vi "M2p_AD+DA_Std_Sync.vi"() -> ()   [LabVIEW 2015]
uses:
  spcm_library/spcm_gui_m2p.llb/element_m2p_ad_std.ctl
  spcm_library/spcm_gui_m2p.llb/element_m2p_ai_channel.ctl
  spcm_library/spcm_gui_common.llb/element_mode.ctl
  spcm_library/spcm_gui_m2p.llb/element_m2p_clock.ctl
  spcm_library/spcm_gui_m2p.llb/element_m2p_ai_trigger.ctl
  spcm_library/spcm_gui_m2p.llb/element_m2p_ai_multi_purpose_io.ctl
  spcm_library/spcm_gui_m2p.llb/element_m2p_da_std.ctl
  spcm_library/spcm_gui_m2p.llb/element_m2p_ao_channel.ctl
  spcm_library/spcm_gui_common.llb/element_mode_out.ctl
  spcm_library/spcm_gui_m2p.llb/element_m2p_ao_trigger.ctl
  spcm_library/spcm_gui_m2p.llb/element_m2p_ao_multi_purpose_io.ctl
  spcm_library/spcm_gui_common.llb/element_devices.ctl
  spcm_library/spcm_gui_common.llb/element_states_io_sync.ctl
panel:
  in  "Waveform":cluster{"Waveform":u16, "Ampl / %":dbl}={"Waveform"=0, "Ampl / %"=100.0} {"Waveform" items=["Sine", "Square", "Ramp"]}
  out "Display Data":sgl[][](graph)
  in  "Devices":T1 {"Device" items=["Card", "digitizerNETBOX"]}
  in  "Tab Control":enum32{"AD Settings", "DA Settings"}(tab)
  in  "Array AD Settings":T2[](array[typedef])=[{"AI Channel 0"={"Enable"=TRUE, "Input Range "=2, "Termination"=0, "Input Type"=0, "Offset"=0}, "AI Channel 1"={"Enable"=TRUE, "Input Range "=2, "Termination"=0, "Input Type"=0, "Offset"=0}, "AI Channel 2"={"Enable"=TRUE, "Input Range "=2, "Termination"=0, "Input Type"=0, "Offset"=0}, "AI Channel 3"={"Enable"=TRUE, "Input Range "=2, "Termination"=0, "Input Type"=0, "Offset"=0}, "AI Channel 4"={"Enable"=TRUE, "Input Range "=2, "Termination"=0, "Input Type"=0, "Offset"=0}, "AI Channel 5"={"Enable"=TRUE, "Input Range "=2, "Termination"=0, "Input Type"=0, "Offset"=0}, "AI Channel 6"={"Enable"=TRUE, "Input Range "=2, "Termination"=0, "Input Type"=0, "Offset"=0}, "AI Channel 7"={"Enable"=TRUE, "Input Range "=2, "Termination"=0, "Input Type"=0, "Offset"=0}, "Mode Setup"={"Mode"=0, "Mem"=16384, "Seg"=1024, "Post"=8192, "Pre"=32, "ABA"=16}, "Clock Settings"={"Clock Mode"=0, "Sampling Rate (kHz)"=10000.0, "Clock Output"=FALSE, "Termination"=FALSE, "Ref. Clock (MHz)"=10.0, "Threshold (mV)"=1500}, "Trigger Settings"={"Trigger Source"=0, "External Trigger"=0, "Level 0 Ext"=1500, "Ext Trig Term"=FALSE, "Channel Trigger"=1, "Level 0 Ch"=0, "Level 1 Ch"=0, "Trigger Delay (Samples)"=0}, "Multi Purpose IO Lines"={"X0 Mode"=0, "X1 Mode"=0, "X2 Mode"=0, "X3 Mode"=0, "X0 ASync Send Pulse"=FALSE, "X1 ASync Send Pulse"=FALSE, "X2 ASync Send Pulse"=FALSE, "X3 ASync Send Pulse"=FALSE, "X1 Trigger Mode"=0, "X2 Trigger Mode"=0, "X3 Trigger Mode"=0, "X1 Pulsewidth"=0, "X2 Pulsewidth"=0, "X3 Pulsewidth"=0, "ASync Read Button"=FALSE, "ASync Read"=0, "AI"=FALSE}}] {"Multi Purpose IO Lines"."X3 Mode" items=["Disable", "Asynchronous Out", "Asynchronous In", "Trigger Out", "Trigger In", "Clock Out", "Digital In", "Show Run State", "Show Arm State", "Show Sync Arm State"]; "Multi Purpose IO Lines"."X2 Mode" items=["Disable", "Asynchronous Out", "Asynchronous In", "Trigger Out", "Trigger In", "Clock Out", "Digital In", "Show Run State", "Show Arm State", "Show Sync Arm State"]; "Multi Purpose IO Lines"."X3 Trigger Mode" items=["Pos. Edge", "Neg. Edge", "Any Edge", "High Level", "Low Level", "PW Long Pos.", "PW Long Neg.", "PW Short Pos.", "PW Short Neg."]; "Multi Purpose IO Lines"."X2 Trigger Mode" items=["Pos. Edge", "Neg. Edge", "Any Edge", "High Level", "Low Level", "PW Long Pos.", "PW Long Neg.", "PW Short Pos.", "PW Short Neg."]; "Multi Purpose IO Lines"."X1 Trigger Mode" items=["Pos. Edge", "Neg. Edge", "Any Edge", "High Level", "Low Level", "PW Long Pos.", "PW Long Neg.", "PW Short Pos.", "PW Short Neg."]; "Multi Purpose IO Lines"."X1 Mode" items=["Disable", "Asynchronous Out", "Asynchronous In", "Trigger Out", "Trigger In", "Clock Out", "Digital In", "Show Run State", "Show Arm State", "Show Sync Arm State"]; "Multi Purpose IO Lines"."X0 Mode" items=["Disable", "Asynchronous Out", "Trigger Out", "Clock Out", "Show Run State", "Show Arm State", "Show Sync Arm State"]; "Trigger Settings"."Channel Trigger" items=["None", "Pos. Edge", "Neg. Edge", "Any Edge", "Pos. Rearm", "Neg. Rearm", "Enter Window", "Leave Window", "In Win", "Out Win"]; "Trigger Settings"."External Trigger" items=["None", "Pos. Edge", "Neg. Edge", "Any Edge", "High Level", "Low Level"]; "Trigger Settings"."Trigger Source" items=["Software Trigger", "External Trigger", "Channel 0 Trigger", "Channel 1 Trigger", "Channel 2 Trigger", "Channel 3 Trigger", "Channel 4 Trigger", "Channel 5 Trigger", "Channel 6 Trigger", "Channel 7 Trigger"]; "Trigger Settings"."Trigger Delay (Samples)" max=65535 step=1; "Clock Settings"."Threshold (mV)" min=-5000 max=5000; "Clock Settings"."Clock Mode" items=["Internal Clock Quartz", "External Clock", "External Reference Clock"]; "Clock Settings"."Ref. Clock (MHz)" min=0.0 max=125000.0; "Clock Settings"."Sampling Rate (kHz)" min=1.0 max=5000000.0; "Mode Setup"."Mode" items=["Singleshot", "Multiple Recording", "Gated Sampling", "ABA Mode"]; "Mode Setup"."ABA" min=2 max=65535 step=1; "Mode Setup"."Post" min=4 step=4; "Mode Setup"."Mem" min=8 step=4; "Mode Setup"."Pre" min=4 max=8176 step=4; "Mode Setup"."Seg" min=8 step=4; "AI Channel 7"."Input Type" items=["Single-ended", "Differential"]; "AI Channel 7"."Termination" items=["1 MOhm", "50 Ohm"]; "AI Channel 7"."Input Range" items=["±200 mV", "±500 mV", "±1000 mV", "±2000 mV", "±5000 mV", "±10000 mV"]; "AI Channel 6"."Input Type" items=["Single-ended", "Differential"]; "AI Channel 6"."Termination" items=["1 MOhm", "50 Ohm"]; "AI Channel 6"."Input Range" items=["±200 mV", "±500 mV", "±1000 mV", "±2000 mV", "±5000 mV", "±10000 mV"]; "AI Channel 5"."Input Type" items=["Single-ended", "Differential"]; "AI Channel 5"."Termination" items=["1 MOhm", "50 Ohm"]; "AI Channel 5"."Input Range" items=["±200 mV", "±500 mV", "±1000 mV", "±2000 mV", "±5000 mV", "±10000 mV"]; "AI Channel 4"."Input Type" items=["Single-ended", "Differential"]; "AI Channel 4"."Termination" items=["1 MOhm", "50 Ohm"]; "AI Channel 4"."Input Range" items=["±200 mV", "±500 mV", "±1000 mV", "±2000 mV", "±5000 mV", "±10000 mV"]; "AI Channel 3"."Input Type" items=["Single-ended", "Differential"]; "AI Channel 3"."Termination" items=["1 MOhm", "50 Ohm"]; "AI Channel 3"."Input Range" items=["±200 mV", "±500 mV", "±1000 mV", "±2000 mV", "±5000 mV", "±10000 mV"]; "AI Channel 2"."Input Type" items=["Single-ended", "Differential"]; "AI Channel 2"."Termination" items=["1 MOhm", "50 Ohm"]; "AI Channel 2"."Input Range" items=["±200 mV", "±500 mV", "±1000 mV", "±2000 mV", "±5000 mV", "±10000 mV"]; "AI Channel 1"."Input Type" items=["Single-ended", "Differential"]; "AI Channel 1"."Termination" items=["1 MOhm", "50 Ohm"]; "AI Channel 1"."Input Range" items=["±200 mV", "±500 mV", "±1000 mV", "±2000 mV", "±5000 mV", "±10000 mV"]; "AI Channel 0"."Input Type" items=["Single-ended", "Differential"]; "AI Channel 0"."Termination" items=["1 MOhm", "50 Ohm"]; "AI Channel 0"."Input Range" items=["±200 mV", "±500 mV", "±1000 mV", "±2000 mV", "±5000 mV", "±10000 mV"]}
  in  "Select AD Device to setup":u16(ring) items=["M2p.5968-x4, SN: 5"]
  in  "Array DA Settings":T8[](array[typedef])=[{"Output Channel 0"={"Enable"=TRUE, "Output Mode"=1, "Gain"=500, "Offset"=0, "Filter"=0, "Stop Level"=0}, "Output Channel 1"={"Enable"=TRUE, "Output Mode"=0, "Gain"=500, "Offset"=0, "Filter"=0, "Stop Level"=0}, "Output Channel 2"={"Enable"=TRUE, "Output Mode"=0, "Gain"=500, "Offset"=0, "Filter"=0, "Stop Level"=0}, "Output Channel 3"={"Enable"=TRUE, "Output Mode"=0, "Gain"=500, "Offset"=0, "Filter"=0, "Stop Level"=0}, "Output Channel 4"={"Enable"=TRUE, "Output Mode"=0, "Gain"=500, "Offset"=0, "Filter"=0, "Stop Level"=0}, "Output Channel 5"={"Enable"=TRUE, "Output Mode"=0, "Gain"=500, "Offset"=0, "Filter"=0, "Stop Level"=0}, "Output Channel 6"={"Enable"=TRUE, "Output Mode"=0, "Gain"=500, "Offset"=0, "Filter"=0, "Stop Level"=0}, "Output Channel 7"={"Enable"=TRUE, "Output Mode"=0, "Gain"=500, "Offset"=0, "Filter"=0, "Stop Level"=0}, "Mode Setup"={"Mode"=1, "Mem"=1024, "Seg"=1024, "Loop"=0}, "Clock Settings"={"Clock Mode"=0, "Sampling Rate (kHz)"=10000.0, "Clock Output"=FALSE, "Termination"=FALSE, "Ref. Clock (MHz)"=10.0, "Threshold (mV)"=1500}, "Trigger Settings"={"Trigger Source"=0, "External Trigger"=0, "TRG_EXT0_LVL0"=1500, "Ext Trig Term"=FALSE, "TRG_EXT0_PW"=1500, "Trigger Delay (samples)"=0}, "Multi Purpose IO Lines"={"X0 Mode"=0, "X1 Mode"=0, "X2 Mode"=0, "X3 Mode"=0, "X0 ASync Send Pulse"=FALSE, "X1 ASync Send Pulse"=FALSE, "X2 ASync Send Pulse"=FALSE, "X3 ASync Send Pulse"=FALSE, "X1 Trigger Mode"=0, "X2 Trigger Mode"=0, "X3 Trigger Mode"=0, "X1 Pulsewidth"=0, "X2 Pulsewidth"=0, "X3 Pulsewidth"=0, "ASync Read Button"=FALSE, "ASync Read"=0, "AI"=FALSE}}] {"Multi Purpose IO Lines"."ASync Read" format="%.0x"; "Multi Purpose IO Lines"."X3 Mode" items=["Disable", "Asynchronous Out", "Asynchronous In", "Trigger Out", "Trigger In", "Clock Out", "Digital Out", "Cont. Output Marker", "Show Run State", "Show Arm State", "Show Sync Arm State"]; "Multi Purpose IO Lines"."X2 Mode" items=["Disable", "Asynchronous Out", "Asynchronous In", "Trigger Out", "Trigger In", "Clock Out", "Digital Out", "Cont. Output Marker", "Show Run State", "Show Arm State", "Show Sync Arm State"]; "Multi Purpose IO Lines"."X3 Trigger Mode" items=["Pos. Edge", "Neg. Edge", "Any Edge", "High Level", "Low Level", "PW Long Pos.", "PW Long Neg.", "PW Short Pos.", "PW Short Neg."]; "Multi Purpose IO Lines"."X2 Trigger Mode" items=["Pos. Edge", "Neg. Edge", "Any Edge", "High Level", "Low Level", "PW Long Pos.", "PW Long Neg.", "PW Short Pos.", "PW Short Neg."]; "Multi Purpose IO Lines"."X1 Trigger Mode" items=["Pos. Edge", "Neg. Edge", "Any Edge", "High Level", "Low Level", "PW Long Pos.", "PW Long Neg.", "PW Short Pos.", "PW Short Neg."]; "Multi Purpose IO Lines"."X1 Mode" items=["Disable", "Asynchronous Out", "Asynchronous In", "Trigger Out", "Trigger In", "Clock Out", "Digital Out", "Cont. Output Marker", "Show Run State", "Show Arm State", "Show Sync Arm State"]; "Multi Purpose IO Lines"."X0 Mode" items=["Disable", "Asynchronous Out", "Trigger Out", "Clock Out", "Digital Out", "Cont. Output Marker", "Show Run State", "Show Arm State", "Show Sync Arm State"]; "Trigger Settings"."External Trigger" items=["None", "Pos. Edge", "Neg. Edge", "Any Edge", "High Level", "Low Level", "PW Long Pos.", "PW Long Neg.", "PW Short Pos.", "PW Short Neg."]; "Trigger Settings"."Trigger Source" items=["Software Trigger", "External Trigger"]; "Trigger Settings"."Trigger Delay (samples)" max=65535 step=1; "Clock Settings"."Threshold (mV)" min=-5000 max=5000; "Clock Settings"."Clock Mode" items=["Internal Clock Quartz", "External Clock", "External Reference Clock"]; "Clock Settings"."Ref. Clock (MHz)" min=0.0 max=125000.0; "Clock Settings"."Sampling Rate (kHz)" min=1.0 max=5000000.0; "Mode Setup"."Mode" items=["Singleshot", "Continuous", "Single Restart", "Multiple Replay", "Gated Replay"]; "Mode Setup"."Loop" step=1; "Mode Setup"."Mem" min=8 step=4; "Mode Setup"."Seg" min=8 step=4; "Output Channel 7"."Filter" items=["Filter 0", "Filter 1", "Filter 2", "Filter 3"]; "Output Channel 7"."Stop Level" items=["Zero", "Low", "High", "Hold Last"]; "Output Channel 7"."Output Mode" items=["Single", "Double", "Differential"]; "Output Channel 6"."Filter" items=["Filter 0", "Filter 1", "Filter 2", "Filter 3"]; "Output Channel 6"."Stop Level" items=["Zero", "Low", "High", "Hold Last"]; "Output Channel 6"."Output Mode" items=["Single", "Double", "Differential"]; "Output Channel 5"."Filter" items=["Filter 0", "Filter 1", "Filter 2", "Filter 3"]; "Output Channel 5"."Stop Level" items=["Zero", "Low", "High", "Hold Last"]; "Output Channel 5"."Output Mode" items=["Single", "Double", "Differential"]; "Output Channel 4"."Filter" items=["Filter 0", "Filter 1", "Filter 2", "Filter 3"]; "Output Channel 4"."Stop Level" items=["Zero", "Low", "High", "Hold Last"]; "Output Channel 4"."Output Mode" items=["Single", "Double", "Differential"]; "Output Channel 3"."Filter" items=["Filter 0", "Filter 1", "Filter 2", "Filter 3"]; "Output Channel 3"."Stop Level" items=["Zero", "Low", "High", "Hold Last"]; "Output Channel 3"."Output Mode" items=["Single", "Double", "Differential"]; "Output Channel 2"."Filter" items=["Filter 0", "Filter 1", "Filter 2", "Filter 3"]; "Output Channel 2"."Stop Level" items=["Zero", "Low", "High", "Hold Last"]; "Output Channel 2"."Output Mode" items=["Single", "Double", "Differential"]; "Output Channel 1"."Filter" items=["Filter 0", "Filter 1", "Filter 2", "Filter 3"]; "Output Channel 1"."Stop Level" items=["Zero", "Low", "High", "Hold Last"]; "Output Channel 1"."Output Mode" items=["Single", "Double", "Differential"]; "Output Channel 0"."Filter" items=["Filter 0", "Filter 1", "Filter 2", "Filter 3"]; "Output Channel 0"."Stop Level" items=["Zero", "Low", "High", "Hold Last"]; "Output Channel 0"."Output Mode" items=["Single", "Double", "Differential"]}
  in  "Select DA Device to setup":u16(ring) items=["M2p.6568-x4, SN: 7"]
  out "Sync Count":u32
  out "Status":string
  in  "Singleshot Button":bool
  in  "Quit Button":bool
  in  "Stop Button":bool
  # "Waveform"
  # "Ampl / %"
  # "Type"
  # "Offset"
  # "Range"
  # "Term"
  # "Mode / Clock / Multi IO"
  # "Trigger"
  # "Mode"
  # "ASync Write"
  # "Trig-Mode"
  # "Trig-Pulsewidth"
  # "ASync Read"
  # "Output Mode"
  # "Offset"
  # "Filter"
  # "Stop Level"
  # "Trigger"
  # "Mode / Clock / Multi IO"
  # "Gain"
  # "Mode"
  # "ASync Write"
  # "Trig-Mode"
  # "Trig-Pulsewidth"
  # "ASync Read"
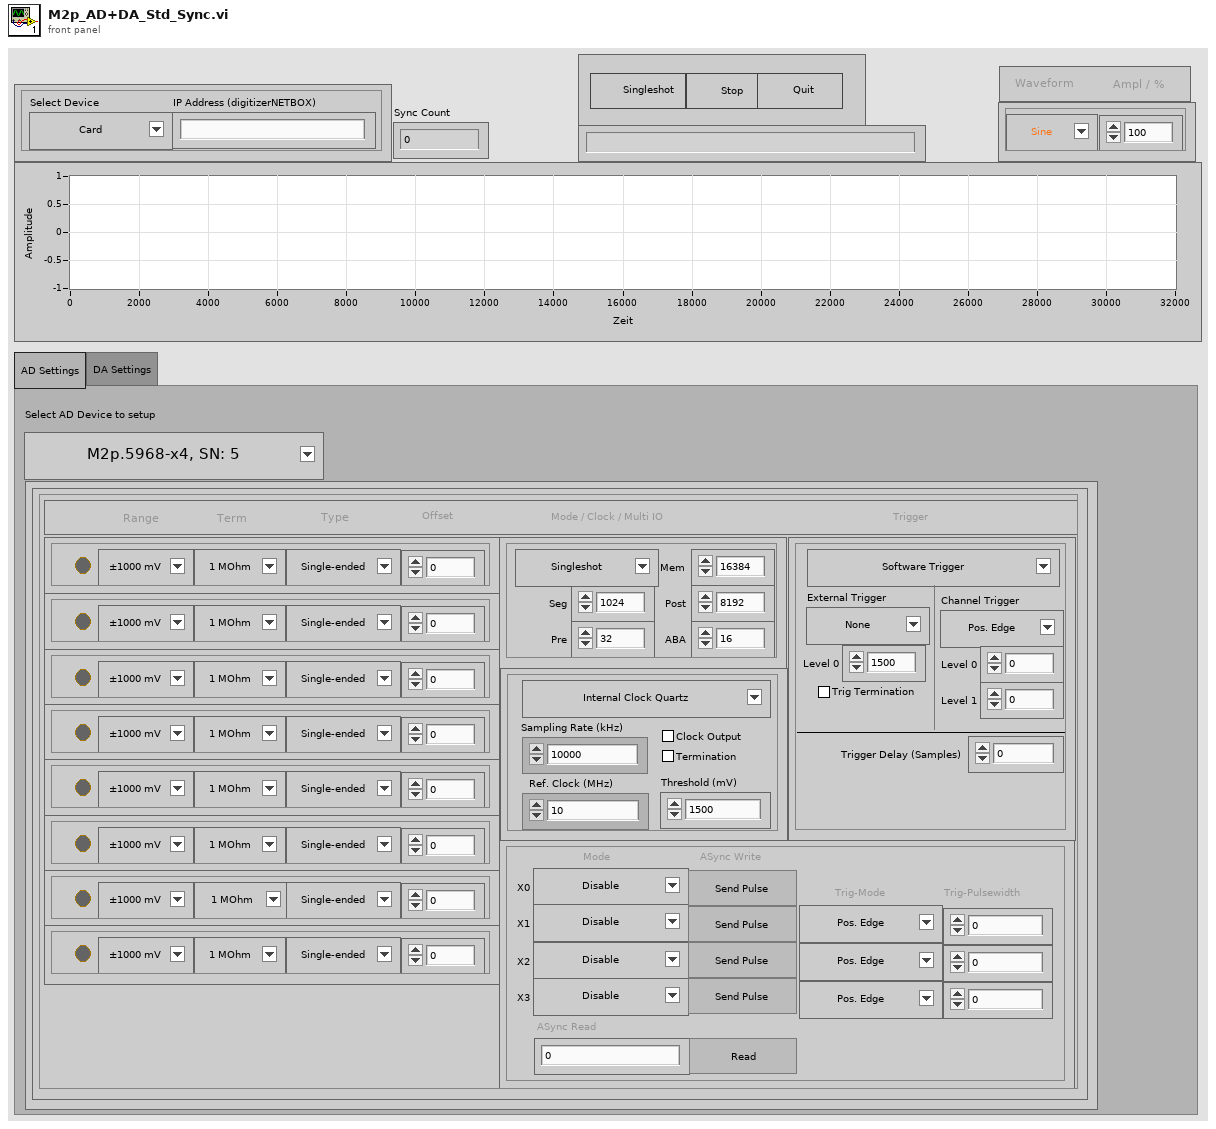
[diagram p1: front panel]
types:
  T1 = typedef "element_devices.ctl" = cluster{"IP Address":string, "Device":u16}
  T2 = typedef "element_m2p_ad_std.ctl" = cluster{"AI Channel 0":T3, "AI Channel 1":T3, "AI Channel 2":T3, "AI Channel 3":T3, "AI Channel 4":T3, "AI Channel 5":T3, "AI Channel 6":T3, "AI Channel 7":T3, "Mode Setup":T4, "Clock Settings":T5, "Trigger Settings":T6, "Multi Purpose IO Lines":T7}
  T3 = typedef "element_m2p_ai_channel.ctl" = cluster{"Enable":bool, "Input Range ":u16, "Termination":u16, "Input Type":u16, "Offset":i32}
  T4 = typedef "element_mode.ctl" = cluster{"Mode":u16, "Mem":u32, "Seg":u32, "Post":u32, "Pre":u32, "ABA":u32}
  T5 = typedef "element_m2p_clock.ctl" = cluster{"Clock Mode":u16, "Sampling Rate (kHz)":dbl, "Clock Output":bool, "Termination":bool, "Ref. Clock (MHz)":dbl, "Threshold (mV)":i32}
  T6 = typedef "element_m2p_ai_trigger.ctl" = cluster{"Trigger Source":u16, "External Trigger":u16, "Level 0 Ext":i32, "Ext Trig Term":bool, "Channel Trigger":u16, "Level 0 Ch":i32, "Level 1 Ch":i32, "Trigger Delay (Samples)":u32}
  T7 = typedef "element_m2p_ai_multi_purpose_io.ctl" = cluster{"X0 Mode":u16, "X1 Mode":u16, "X2 Mode":u16, "X3 Mode":u16, "X0 ASync Send Pulse":bool, "X1 ASync Send Pulse":bool, "X2 ASync Send Pulse":bool, "X3 ASync Send Pulse":bool, "X1 Trigger Mode":u16, "X2 Trigger Mode":u16, "X3 Trigger Mode":u16, "X1 Pulsewidth":u32, "X2 Pulsewidth":u32, "X3 Pulsewidth":u32, "ASync Read Button":bool, "ASync Read":i32, "AI":bool}
  T8 = typedef "element_m2p_da_std.ctl" = cluster{"Output Channel 0":T9, "Output Channel 1":T9, "Output Channel 2":T9, "Output Channel 3":T9, "Output Channel 4":T9, "Output Channel 5":T9, "Output Channel 6":T9, "Output Channel 7":T9, "Mode Setup":T10, "Clock Settings":T5, "Trigger Settings":T11, "Multi Purpose IO Lines":T12}
  T9 = typedef "element_m2p_ao_channel.ctl" = cluster{"Enable":bool, "Output Mode":u16, "Gain":i32, "Offset":i32, "Filter":u16, "Stop Level":u16}
  T10 = typedef "element_mode_out.ctl" = cluster{"Mode":u16, "Mem":u32, "Seg":u32, "Loop":u32}
  T11 = typedef "element_m2p_ao_trigger.ctl" = cluster{"Trigger Source":u16, "External Trigger":u16, "TRG_EXT0_LVL0":i32, "Ext Trig Term":bool, "TRG_EXT0_PW":i32, "Trigger Delay (samples)":u32}
  T12 = typedef "element_m2p_ao_multi_purpose_io.ctl" = cluster{"X0 Mode":u16, "X1 Mode":u16, "X2 Mode":u16, "X3 Mode":u16, "X0 ASync Send Pulse":bool, "X1 ASync Send Pulse":bool, "X2 ASync Send Pulse":bool, "X3 ASync Send Pulse":bool, "X1 Trigger Mode":u16, "X2 Trigger Mode":u16, "X3 Trigger Mode":u16, "X1 Pulsewidth":u32, "X2 Pulsewidth":u32, "X3 Pulsewidth":u32, "ASync Read Button":bool, "ASync Read":i32, "AI":bool}
  T13 = typedef "element_states_io_sync.ctl" = enum16{"Idle", "Init GUI", "Init Cards", "Init Sync", "Write Setup", "Write Data", "Start", "Acquire", "Read Data", "Stop", "Close Sync", "Close Cards", "Quit"}
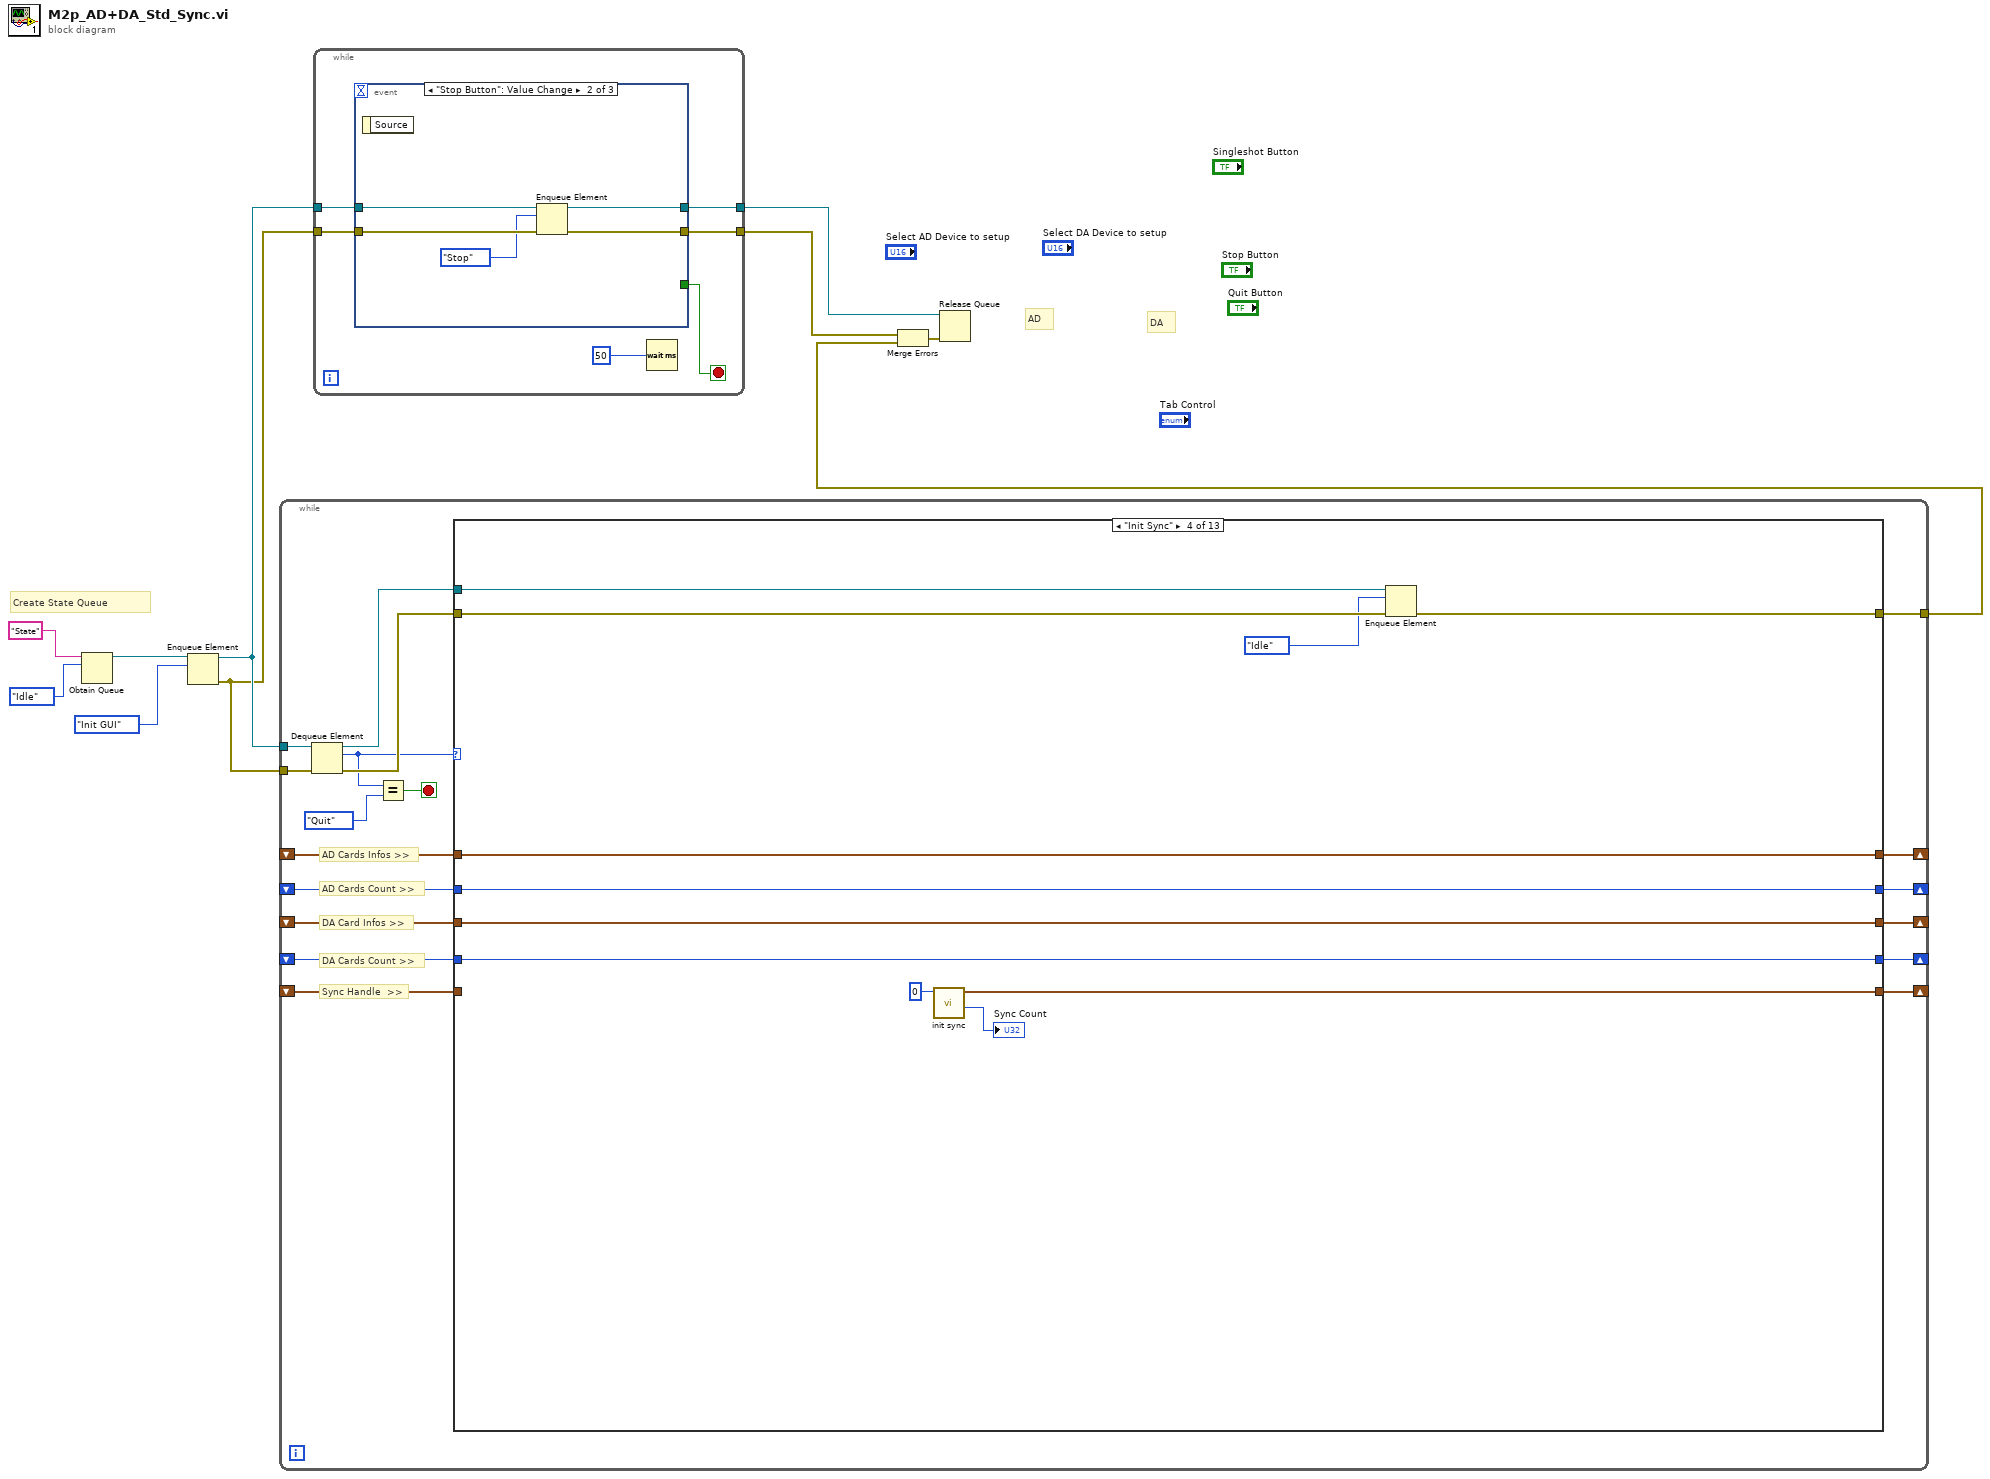
[diagram p0: block diagram]
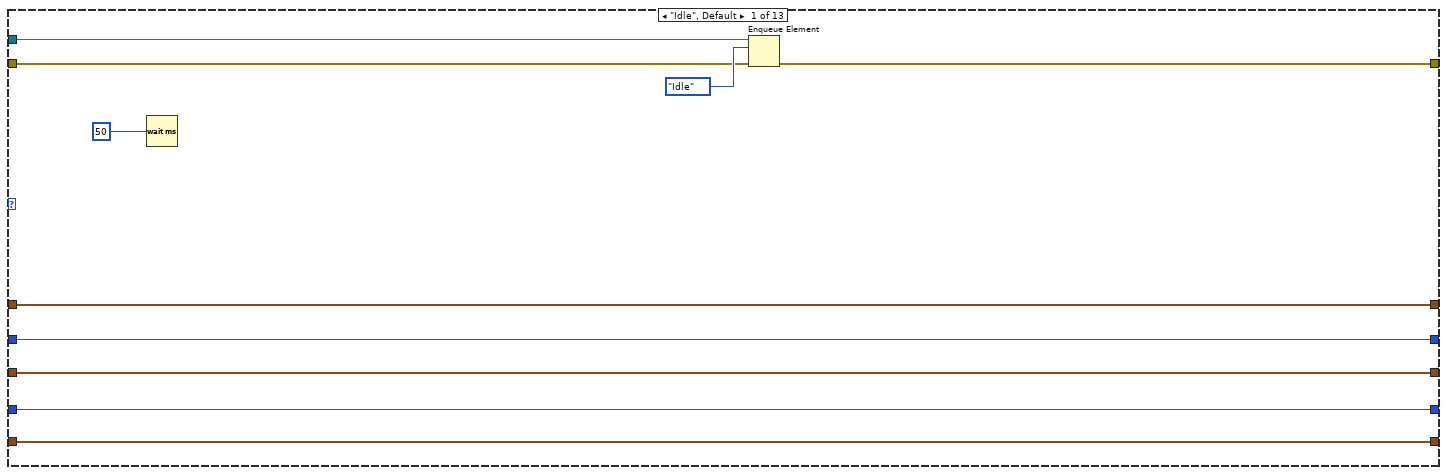
[diagram p2: hidden frame]
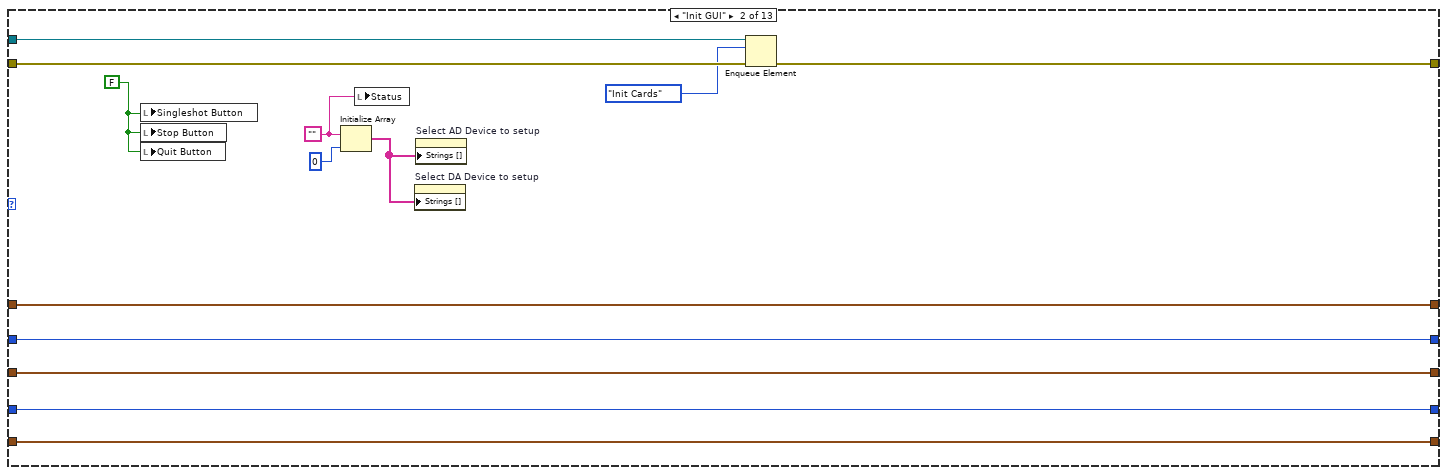
[diagram p3: hidden frame]
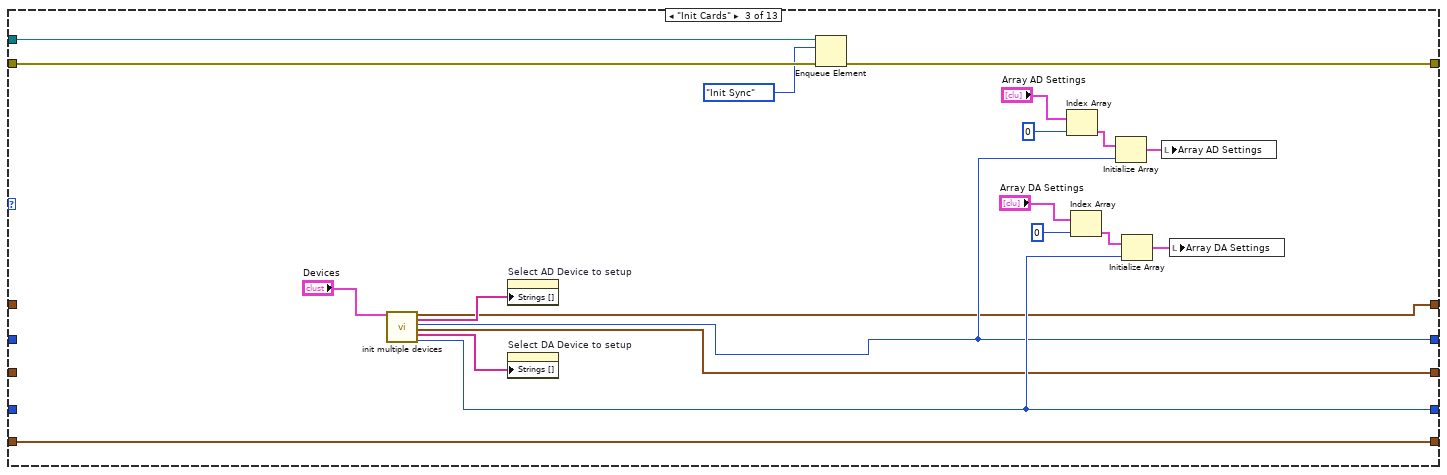
[diagram p4: hidden frame]
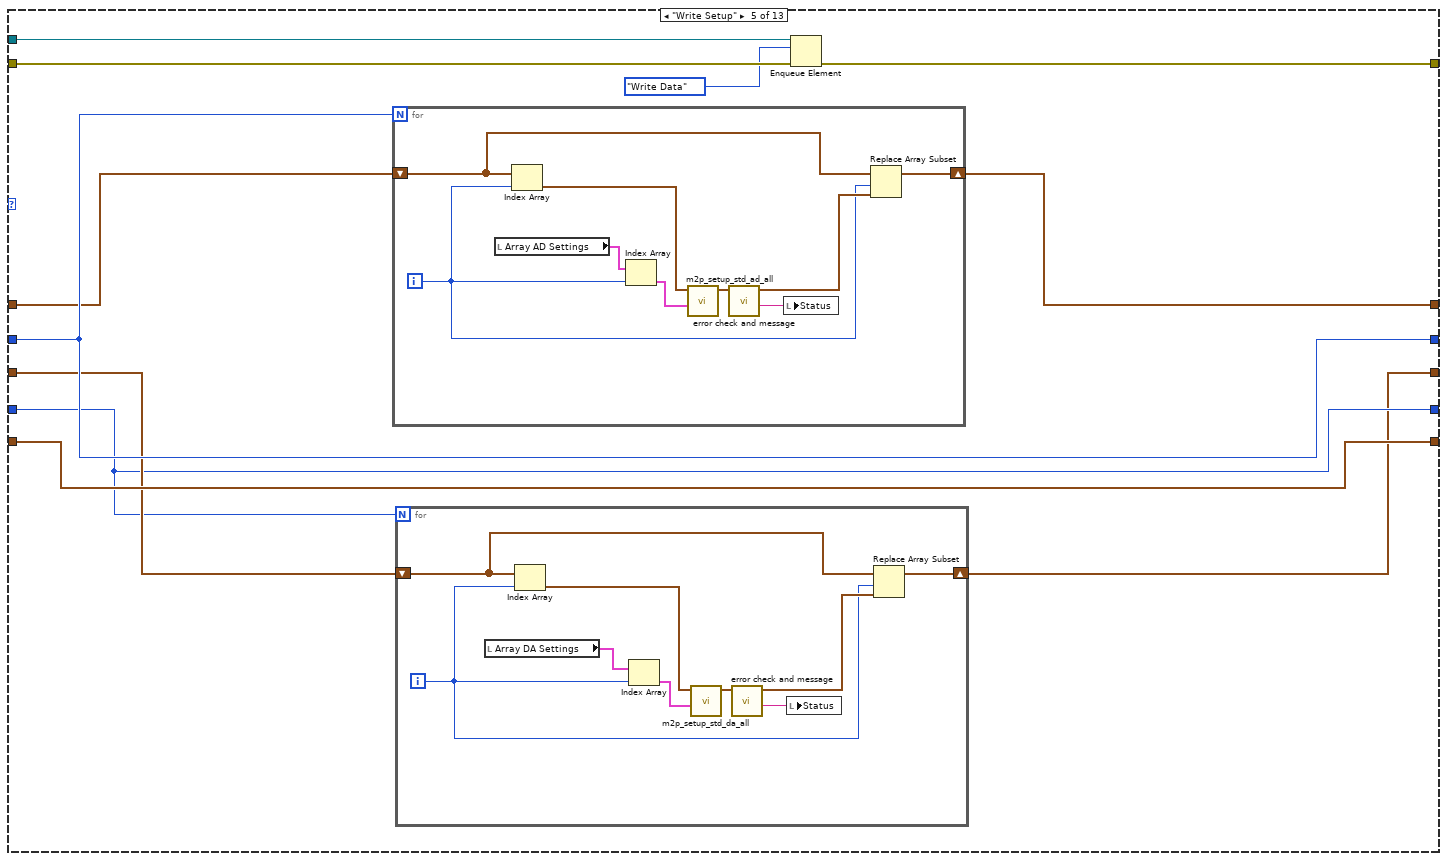
[diagram p5: hidden frame]
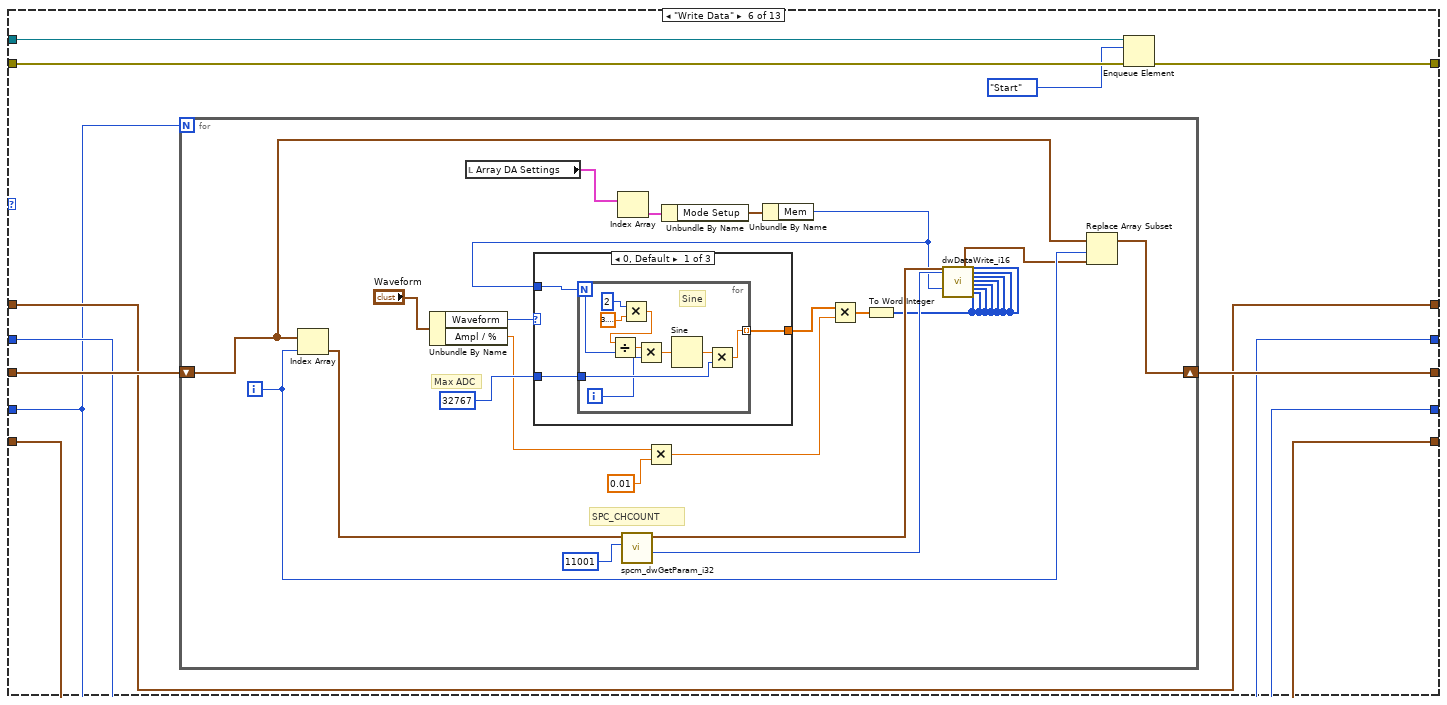
[diagram p6: hidden frame]
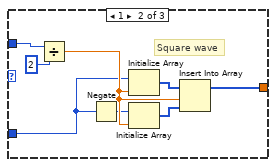
[diagram p7: hidden frame]
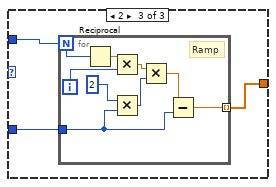
[diagram p8: hidden frame]
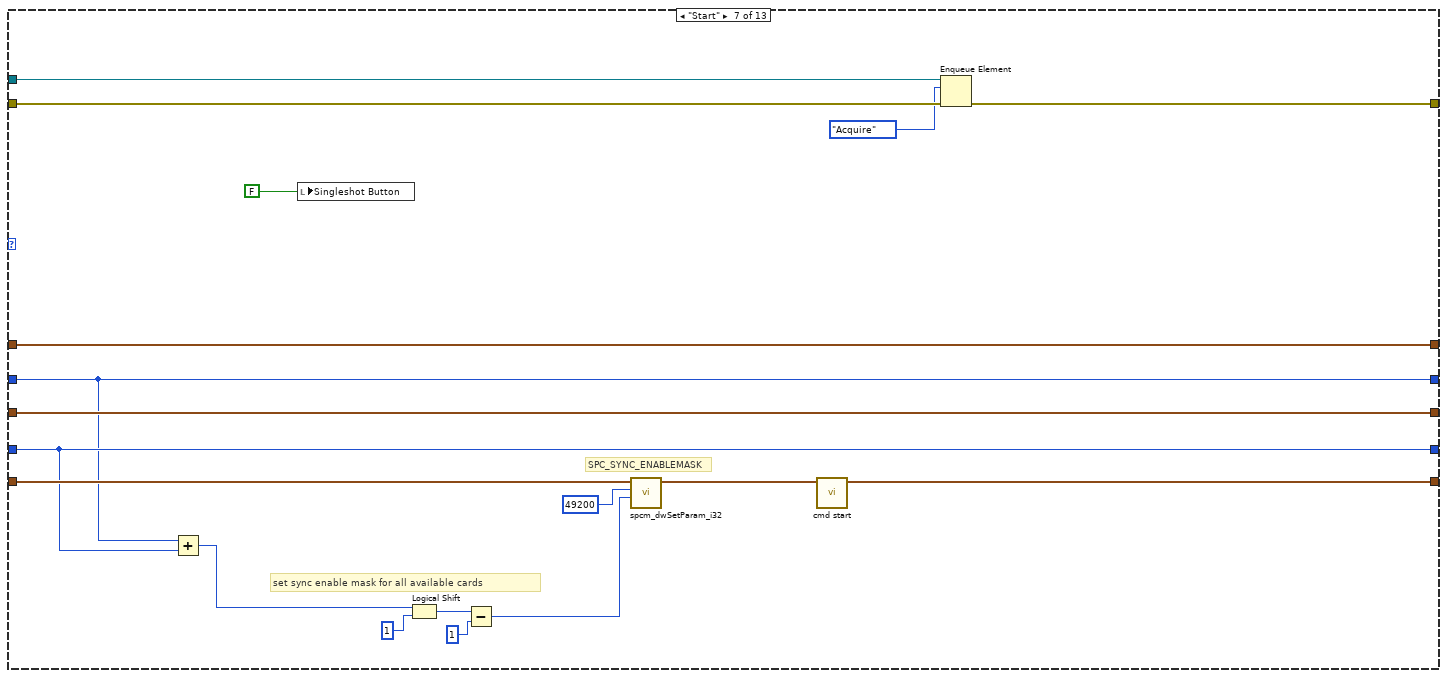
[diagram p9: hidden frame]
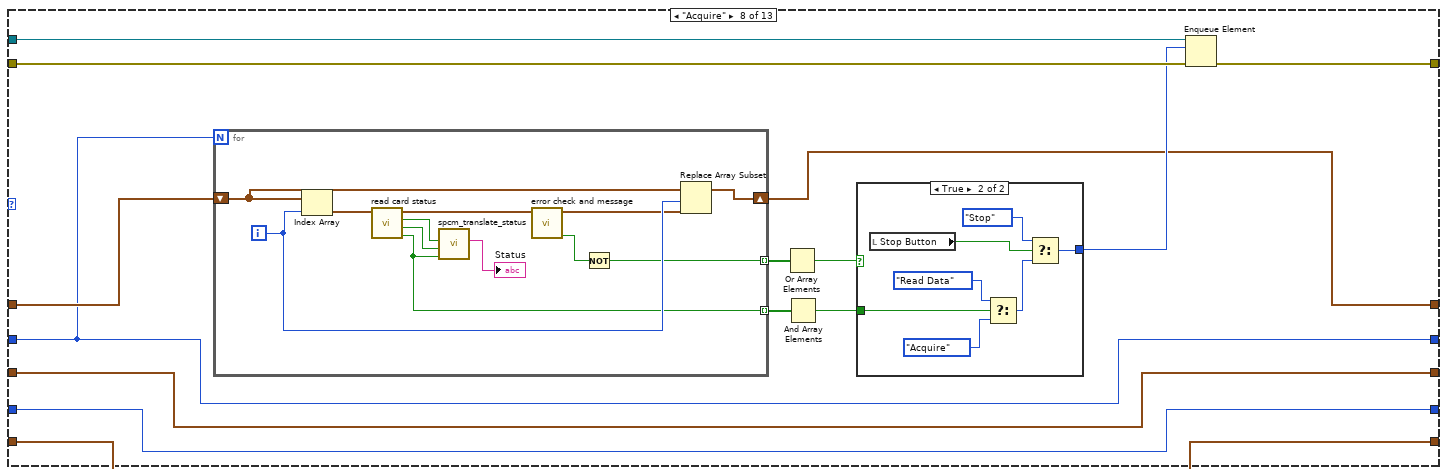
[diagram p10: hidden frame]
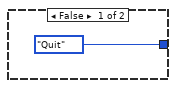
[diagram p11: hidden frame]
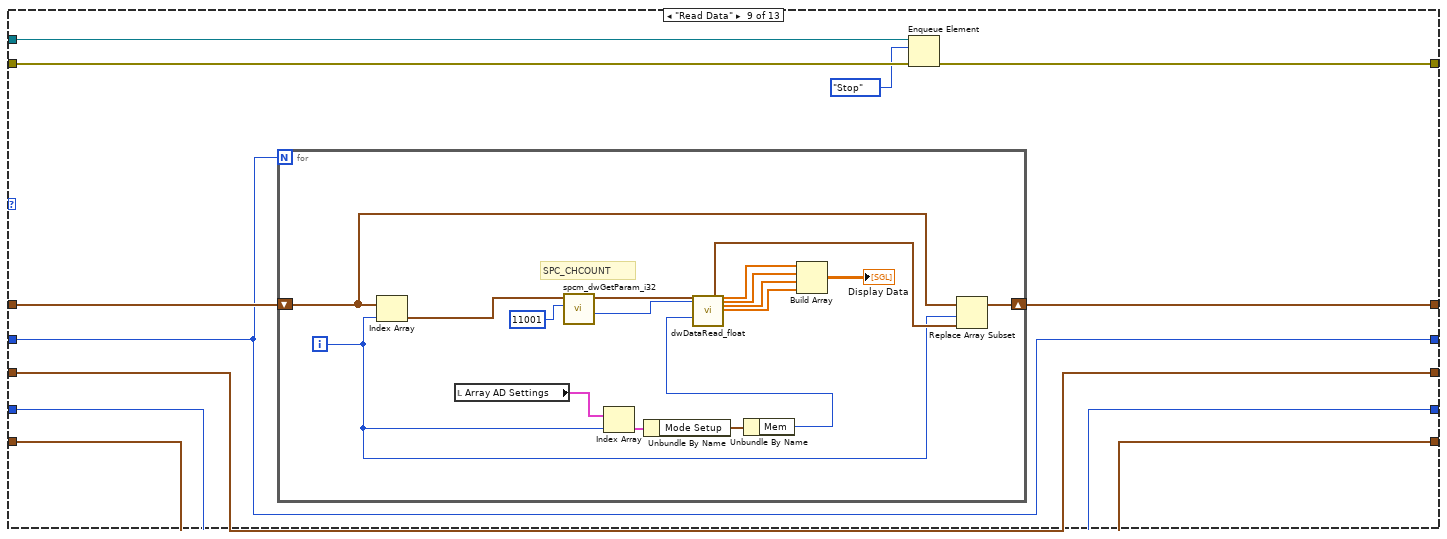
[diagram p12: hidden frame]
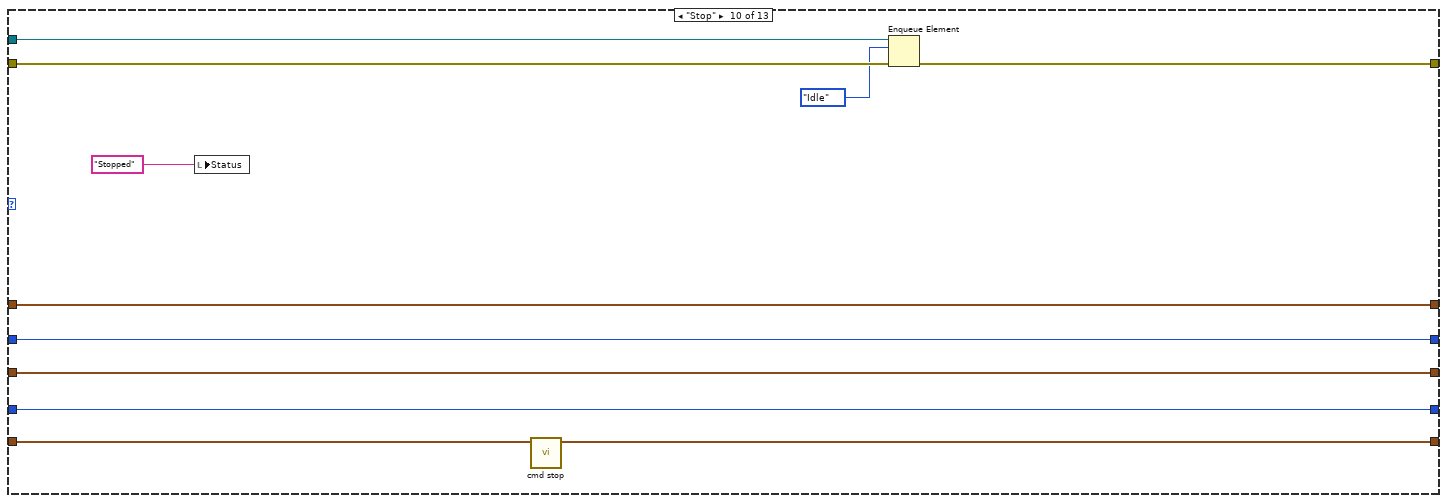
[diagram p13: hidden frame]
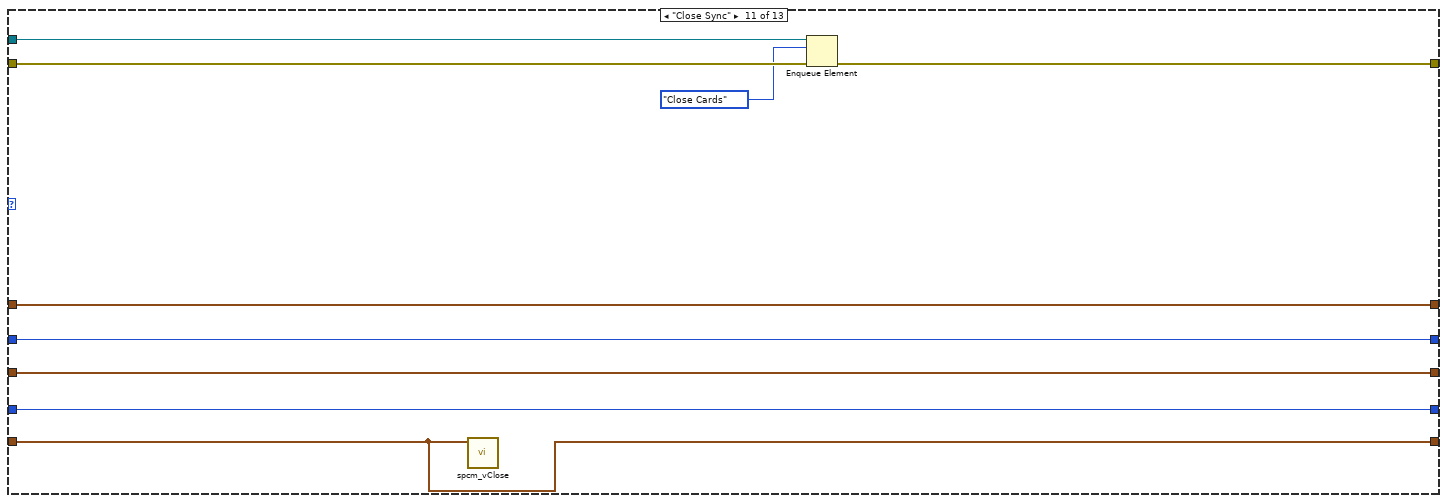
[diagram p14: hidden frame]
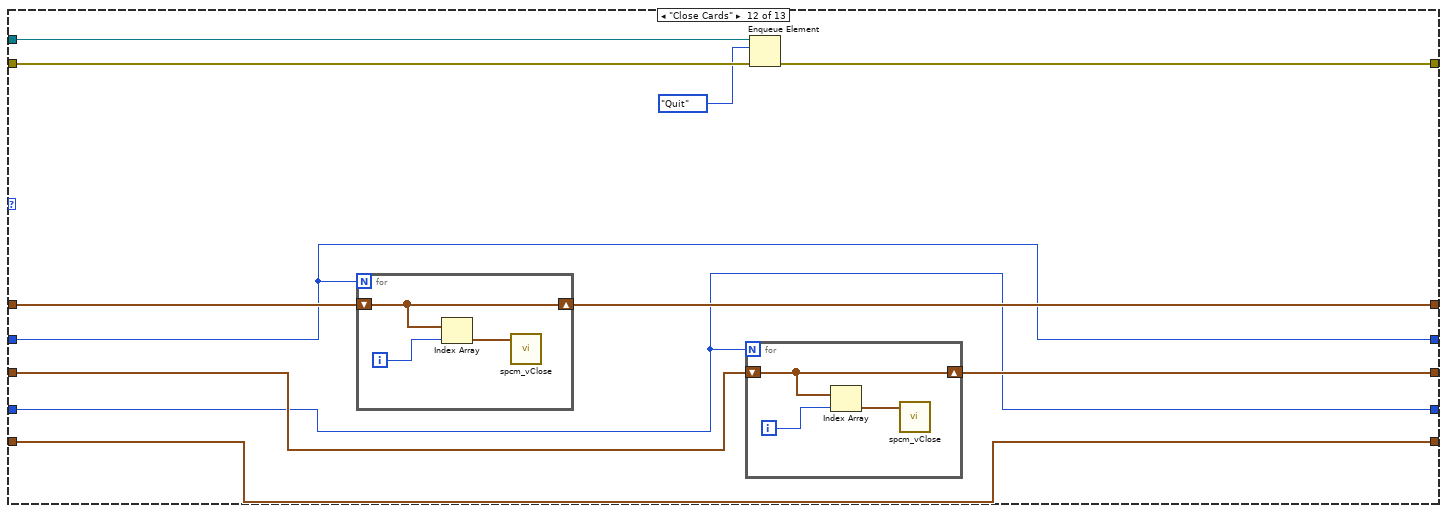
[diagram p15: hidden frame]
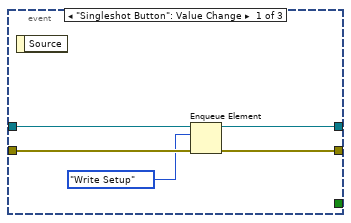
[diagram p17: hidden frame]
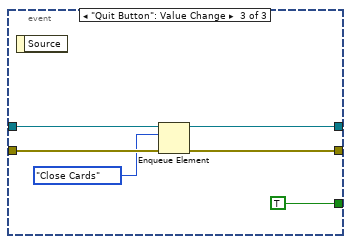
[diagram p18: hidden frame]
diagram:
  # "Create State Queue"
  # "AD"
  # "DA"
  n1 = Obtain Queue(name (unnamed)="State", element data type=element_states_io_sync."Idle") -> (queue out=w8:refnum<queue>)  [unwired: 3 in, 2 out]
  n2 = Enqueue Element(queue=w8, element=element_states_io_sync."Init GUI") -> (queue out=w5:refnum<queue>, error out=w3:errorcluster)  [unwired: 2 in, 1 out]
  n3 = while {
    tunnel: w3 -> [w27]
    tunnel: w5 -> [w28]
    tunnel: [w23] -> w1
    shift-right: [w20] -> _
    shift-left: _ -> [w19]
    shift-right: [w11] -> _
    shift-left: _ -> [w12]
    shift-right: [w13] -> _
    shift-left: _ -> [w18]
    shift-right: [w17] -> _
    shift-left: _ -> [w15]
    shift-right: [w16] -> _
    shift-left: _ -> [w14]
    stop <- w26 stop-if-true
    # "Sync Handle  >>"
    # "DA Cards Count >>"
    # "DA Card Infos >>"
    # "AD Cards Count >>"
    # "AD Cards Infos >>"
    n4 = Dequeue Element(queue=w28, error in (no error)=w27) -> (queue out=w25:refnum<queue>, element=w21:T13, error out=w24:errorcluster)  [unwired: 1 in, 1 out]
    n5 = Equal?(x=w21, y=element_states_io_sync."Quit") -> (x = y?=w26:bool)
    n6 = case shown="\"Init Sync\"" w21 {
      tunnel: w25 -> [w37 w51 w71 w78 w93 w121 w186 w207 w237 w263 w272 w285 _]
      tunnel: w24 -> [w36 w50 w70 w77 w92 w120 w185 w206 w236 w262 w271 w284 w297]
      tunnel: [w34 w49 w68 w76 w91 w118 w184 w205 w235 w261 w269 w283 w297] -> w23
      tunnel: [w33 w43 w53 w80 w84 w115 w193 w198 w232 w265 w274 w281 w296] -> w20
      tunnel: [w32 w42 w54 w79 w89 w114 w178 w197 w231 w264 w273 w276 w295] -> w11
      tunnel: w19 -> [w33 w43 _ w80 w88 w115 w193 w204 w233 w265 w274 w280 w296]
      tunnel: w12 -> [w32 w42 _ w79 w89 w114 w178 w197 w231 w264 w273 w276 w295]
      tunnel: w18 -> [w29 w40 _ w73 w86 w117 w180 w196 w230 w256 w268 w278 w292]
      tunnel: [w31 w41 w55 w72 w85 w113 w179 w195 w229 w257 w267 w275 w294] -> w17
      tunnel: [w30 w39 w64 w74 w87 w112 w176 w194 w228 w258 w266 w277 w293] -> w16
      tunnel: w15 -> [w31 w41 _ w72 w85 w113 w179 w195 w229 w257 w267 w275 w294]
      tunnel: w14 -> [w30 w39 w64 _ w87 w112 w181 w194 w228 w259 w266 w277 w293]
      tunnel: [w29 w40 w52 w73 w83 w116 w180 w196 w230 w256 w268 w279 w292] -> w13
      frame "Idle", Default {
        n7 = Wait (ms)(milliseconds to wait=50) -> ()  [unwired: 1 out]
        n8 = Enqueue Element(queue=w37, element=element_states_io_sync."Idle", error in (no error)=w36) -> (error out=w34:errorcluster)  [unwired: 1 in, 2 out]
      }
      frame "Init GUI" {
        w45 = FALSE
        w44 = ""
        n9 = local write "Singleshot Button"(w45) -> ()
        n10 = local write "Stop Button"(w45) -> ()
        n11 = local write "Quit Button"(w45) -> ()
        n12 = Initialize Array(w44, 0) -> (w46:string[])
        n13 = local write "Status"(w44) -> ()
        n14 = property on="Select DA Device to setup" class="Ring (strict)"("Strings []"=w46) -> ()  [unwired: 2 in, 2 out]
        n15 = property on="Select AD Device to setup" class="Ring (strict)"("Strings []"=w46) -> ()  [unwired: 2 in, 2 out]
        n16 = Enqueue Element(queue=w51, element=element_states_io_sync."Init Cards", error in (no error)=w50) -> (error out=w49:errorcluster)  [unwired: 1 in, 2 out]
      }
      frame "Init Cards" {
        n17 = call "init multiple devices.vi"("Device"="Devices") -> ("AD CardInfos"=w53:cluster{"Card Handle":u64, "Error Code":u32}[], "AD Card Names"=w67:string[], "AD Cards Count"=w54:i32, "DA CardInfos"=w52:cluster{"Card Handle":u64, "Error Code":u32}[], "DA Card Names"=w66:string[], "DA Cards Count"=w55:i32)  [unwired: 13 in]
        n18 = property on="Select AD Device to setup" class="Ring (strict)"("Strings []"=w67) -> ()  [unwired: 2 in, 2 out]
        n19 = property on="Select DA Device to setup" class="Ring (strict)"("Strings []"=w66) -> ()  [unwired: 2 in, 2 out]
        n20 = Enqueue Element(queue=w71, element=element_states_io_sync."Init Sync", error in (no error)=w70) -> (error out=w68:errorcluster)  [unwired: 1 in, 2 out]
        n21 = Index Array(array="Array AD Settings", index=0) -> (element=w63:T2)
        n22 = Index Array(array="Array DA Settings", index=0) -> (element=w59:T8)
        n23 = Initialize Array(w63, w54) -> (w60:T2[])
        n24 = Initialize Array(w59, w55) -> (w56:T8[])
        n25 = local write "Array AD Settings"(w60) -> ()
        n26 = local write "Array DA Settings"(w56) -> ()
      }
      frame "Init Sync" {
        n27 = call "init sync.vi"("Sync Index"=u32 0 ("Card Index")) -> ("Sync count"=→"Sync Count":i32, "Sync Info Out"=w74:cluster{"Sync Handle":u64, "Error Code":u32})  [unwired: 5 in]
        n28 = Enqueue Element(queue=w78, element=element_states_io_sync."Idle", error in (no error)=w77) -> (error out=w76:errorcluster)  [unwired: 1 in, 2 out]
      }
      frame "Write Setup" {
        n29 = for {
          N: w89 -> [_]
          shift-right: [w103] -> w84
          shift-left: w88 -> [w104]
          i -> [w105]
          n30 = local read "Array AD Settings"() -> (w111:T2[])
          n31 = Index Array(array=w104, index=w105) -> (element=w107:cluster{"Card Handle":u64, "Error Code":u32})
          n32 = Index Array(array=w111, index=w105) -> (element=w108:T2)
          n33 = call "m2p_setup_std_ad_all.vi"("Card Info In"=w107, "M2p AD Settings"=w108) -> ("Card Info Out"=w110:cluster{"Card Handle":u64, "Error Code":u32})  [unwired: 4 in, 3 out]
          n34 = call "error check and message.vi"("Card Info In"=w110) -> ("Error Message"=w109:string, "Card Info Out"=w106:cluster{"Card Handle":u64, "Error Code":u32})  [unwired: 4 in, 1 out]
          n35 = local write "Status"(w109) -> ()
          n36 = Replace Array Subset(array=w104, new element=w106, index=w105) -> (w103:cluster{"Card Handle":u64, "Error Code":u32}[])
        }
        n37 = for {
          N: w85 -> [_]
          shift-right: [w98] -> w83
          shift-left: w86 -> [w99]
          i -> [w100]
          n38 = local read "Array DA Settings"() -> (w96:T8[])
          n39 = Index Array(array=w99, index=w100) -> (element=w95:cluster{"Card Handle":u64, "Error Code":u32})
          n40 = Index Array(array=w96, index=w100) -> (element=w94:T8)
          n41 = call "m2p_setup_std_da_all.vi"("M2p DA Settings"=w94, "Card Info In"=w95) -> ("Card Info Out"=w97:cluster{"Card Handle":u64, "Error Code":u32})  [unwired: 6 in, 3 out]
          n42 = call "error check and message.vi"("Card Info In"=w97) -> ("Error Message"=w102:string, "Card Info Out"=w101:cluster{"Card Handle":u64, "Error Code":u32})  [unwired: 4 in, 1 out]
          n43 = local write "Status"(w102) -> ()
          n44 = Replace Array Subset(array=w99, new element=w101, index=w100) -> (w98:cluster{"Card Handle":u64, "Error Code":u32}[])
        }
        n45 = Enqueue Element(queue=w93, element=element_states_io_sync."Write Data", error in (no error)=w92) -> (error out=w91:errorcluster)  [unwired: 1 in, 2 out]
      }
      frame "Write Data" {
        n46 = for {
          N: w113 -> [_]
          shift-right: [w122] -> w116
          shift-left: w117 -> [w123]
          i -> [w125]
          # "SPC_CHCOUNT"
          # "Max ADC"
          n47 = Index Array(array=w123, index=w125) -> (element=w126:cluster{"Card Handle":u64, "Error Code":u32})
          n48 = Unbundle By Name("Waveform") -> ("Waveform"=w135:u16, "Ampl / %"=w131:dbl)
          n49 = local read "Array DA Settings"() -> (w142:T8[])
          n50 = Index Array(array=w142) -> (element=w141:T8)  [unwired: 1 in]
          n51 = call "spcm_dwGetParam_i32.vi"("Register"=11001, "Card Info In"=w126) -> ("Value (int32)"=w137:i32, "Card Info Out"=w138:cluster{"Card Handle":u64, "Error Code":u32})  [unwired: 4 in]
          n52 = Multiply(x=w131, y=0.01) -> (x*y=w128:dbl)
          n53 = Unbundle By Name(w141) -> ("Mode Setup"=w140:T10)
          n54 = Unbundle By Name(w140) -> ("Mem"=w133:u32)
          n55 = case shown="0, Default" w135 {
            tunnel: w133 -> [w143 w163 w166]
            tunnel: [w145 w159 w165] -> w129
            tunnel: 32767 -> [w144 w156 w164]
            frame 0, Default {
              n56 = for {
                N: w143 -> [w148]
                tunnel: [w146] -> w145 mode=indexing
                tunnel: w144 -> [w154]
                i -> [w149]
                # "Sine"
                n57 = Multiply(x=2, y=3.141592653589793) -> (x*y=w147:dbl)
                n58 = Divide(x=w147, y=w148) -> (x/y=w150:dbl)
                n59 = Multiply(x=w150, y=w149) -> (x*y=w151:dbl)
                n60 = Sine(x=w151) -> (sin(x)=w155:dbl)
                n61 = Multiply(x=w155, y=w154) -> (x*y=w146:dbl)
              }
            }
            frame 1 {
              # "Square wave"
              n62 = Divide(x=w163, y=2) -> (x/y=w158:dbl)
              n63 = Negate(x=w156) -> (-x=w157:i32)
              n64 = Initialize Array(w156, w158) -> (w161:i32[])
              n65 = Initialize Array(w157, w158) -> (w160:i32[])
              n66 = Insert Into Array(array=w161, index=w158, new element=w160) -> (w159:i32[])
            }
            frame 2 {
              n67 = for {
                N: w166 -> [w171]
                tunnel: [w173] -> w165 mode=indexing
                tunnel: w164 -> [w167]
                i -> [w175]
                # "Ramp"
                n68 = Reciprocal(x=w171) -> (1/x=w170:dbl)
                n69 = Multiply(x=w170, y=w175) -> (x*y=w174:dbl)
                n70 = Multiply(x=2, y=w167) -> (x*y=w169:i32)
                n71 = Multiply(x=w174, y=w169) -> (x*y=w172:dbl)
                n72 = Subtract(x=w172, y=w167) -> (x-y=w173:dbl)
              }
            }
          }
          n73 = Multiply(x=w129, y=w128) -> (x*y=w130:dbl[])
          n74 = To Word Integer(number=w130) -> (16bit integer=w136:i16[])
          n75 = call "dwDataWrite_i16.vi"("Card Info In"=w138, "Channel Count"=w137, "Length (Samples per Channel)"=w133, "Ch 0"=w136, "Ch 1"=w136, "Ch 2"=w136, "Ch 3"=w136, "Ch 4"=w136, "Ch 5"=w136, "Ch 6"=w136, "Ch 7"=w136) -> ("Card Info Out"=w124:cluster{"Card Handle":u64, "Error Code":u32})  [unwired: 16 in]
          n76 = Replace Array Subset(array=w123, new element=w124, index=w125) -> (w122:cluster{"Card Handle":u64, "Error Code":u32}[])
        }
        n77 = Enqueue Element(queue=w121, element=element_states_io_sync."Start", error in (no error)=w120) -> (error out=w118:errorcluster)  [unwired: 1 in, 2 out]
      }
      frame "Start" {
        # "SPC_SYNC_ENABLEMASK"
        # "set sync enable mask for all available cards"
        n78 = Add(x=w178, y=w179) -> (x+y=w177:i32)
        n79 = local write "Singleshot Button"(FALSE) -> ()
        n80 = Logical Shift(y=w177, x=1) -> (x << y=w191:i32)
        n81 = Subtract(x=w191, y=1) -> (x-y=w188:i32)
        n82 = call "spcm_dwSetParam_i32.vi"("Value (int32)"=w188, "Register"=49200, "Card Info In"=w181) -> ("Card Info Out"=w187:cluster{"Card Handle":u64, "Error Code":u32})  [unwired: 4 in]
        n83 = call "cmd start.vi"("Card Info In"=w187) -> ("Card Info Out"=w176:cluster{"Card Handle":u64, "Error Code":u32})  [unwired: 6 in]
        n84 = Enqueue Element(queue=w186, element=element_states_io_sync."Acquire", error in (no error)=w185) -> (error out=w184:errorcluster)  [unwired: 1 in, 2 out]
      }
      frame "Acquire" {
        n85 = for {
          N: w197 -> [_]
          shift-right: [w221] -> w198
          shift-left: w204 -> [w220]
          tunnel: [w217] -> w202 mode=indexing
          tunnel: [w216] -> w203 mode=indexing
          i -> [w219]
          n86 = Index Array(array=w220, index=w219) -> (element=w222:cluster{"Card Handle":u64, "Error Code":u32})
          n87 = call "read card status.vi"("Card Info In"=w222) -> ("Card ready"=w216:bool, "Trigger detected"=w224:bool, "Pretrigger full"=w225:bool, "Card Info Out"=w226:cluster{"Card Handle":u64, "Error Code":u32})  [unwired: 3 in]
          n88 = call "spcm_translate_status.vi"("Ready"=w216, "Trigger"=w224, "Pretrigger"=w225) -> ("Text"=→"Status":string)  [unwired: 4 in]
          n89 = call "error check and message.vi"("Card Info In"=w226) -> ("Error occurred"=w227:bool, "Card Info Out"=w218:cluster{"Card Handle":u64, "Error Code":u32})  [unwired: 4 in, 1 out]
          n90 = Not(x=w227) -> (.not. x?=w217:bool)
          n91 = Replace Array Subset(array=w220, new element=w218, index=w219) -> (w221:cluster{"Card Handle":u64, "Error Code":u32}[])
        }
        n92 = Or Array Elements(Boolean array=w202) -> (logical OR=w200:bool)
        n93 = And Array Elements(Boolean array=w203) -> (logical AND=w201:bool)
        n94 = case shown="True" w200 {
          tunnel: w201 -> [_ w211]
          tunnel: [element_states_io_sync."Quit" w209] -> w199
          frame False {
          }
          frame True {
            n95 = local read "Stop Button"() -> (w210:bool)
            n96 = Select(t=element_states_io_sync."Read Data", s=w211, f=element_states_io_sync."Acquire") -> (s? t:f=w214:T13)
            n97 = Select(t=element_states_io_sync."Stop", s=w210, f=w214) -> (s? t:f=w209:T13)
          }
        }
        n98 = Enqueue Element(queue=w207, element=w199, error in (no error)=w206) -> (error out=w205:errorcluster)  [unwired: 1 in, 2 out]
      }
      frame "Read Data" {
        n99 = for {
          N: w231 -> [_]
          shift-right: [w238] -> w232
          shift-left: w233 -> [w240]
          i -> [w239]
          # "SPC_CHCOUNT"
          n100 = Index Array(array=w240, index=w239) -> (element=w242:cluster{"Card Handle":u64, "Error Code":u32})
          n101 = local read "Array AD Settings"() -> (w244:T2[])
          n102 = call "spcm_dwGetParam_i32.vi"("Register"=11001, "Card Info In"=w242) -> ("Value (int32)"=w248:i32, "Card Info Out"=w247:cluster{"Card Handle":u64, "Error Code":u32})  [unwired: 4 in]
          n103 = Index Array(array=w244, index=w239) -> (element=w245:T2)
          n104 = Unbundle By Name(w245) -> ("Mode Setup"=w246:T4)
          n105 = Unbundle By Name(w246) -> ("Mem"=w254:u32)
          n106 = call "dwDataRead_float.vi"("Card Info In"=w247, "Channel Count"=w248, "Length (Samples per Channel)"=w254) -> ("Card Info Out"=w241:cluster{"Card Handle":u64, "Error Code":u32}, "Ch 0"=w249:sgl[], "Ch 1"=w250:sgl[], "Ch 2"=w251:sgl[], "Ch 3"=w252:sgl[])  [unwired: 8 in, 12 out]
          n107 = Build Array(w249, w250, w251, w252) -> (→"Display Data":sgl[][])
          n108 = Replace Array Subset(array=w240, new element=w241, index=w239) -> (w238:cluster{"Card Handle":u64, "Error Code":u32}[])
        }
        n109 = Enqueue Element(queue=w237, element=element_states_io_sync."Stop", error in (no error)=w236) -> (error out=w235:errorcluster)  [unwired: 1 in, 2 out]
      }
      frame "Stop" {
        n110 = local write "Status"("Stopped") -> ()
        n111 = call "cmd stop.vi"("Card Info In"=w259) -> ("Card Info Out"=w258:cluster{"Card Handle":u64, "Error Code":u32})  [unwired: 6 in]
        n112 = Enqueue Element(queue=w263, element=element_states_io_sync."Idle", error in (no error)=w262) -> (error out=w261:errorcluster)  [unwired: 1 in, 2 out]
      }
      frame "Close Sync" {
        n113 = call "spcm_vClose.vi"("Card Info In"=w266) -> ()  [unwired: 7 in]
        n114 = Enqueue Element(queue=w272, element=element_states_io_sync."Close Cards", error in (no error)=w271) -> (error out=w269:errorcluster)  [unwired: 1 in, 2 out]
      }
      frame "Close Cards" {
        n115 = for {
          N: w276 -> [_]
          shift-right: [w290] -> w281
          shift-left: w280 -> [w290]
          i -> [w291]
          n116 = Index Array(array=w290, index=w291) -> (element=w289:cluster{"Card Handle":u64, "Error Code":u32})
          n117 = call "spcm_vClose.vi"("Card Info In"=w289) -> ()  [unwired: 7 in]
        }
        n118 = for {
          N: w275 -> [_]
          shift-right: [w287] -> w279
          shift-left: w278 -> [w287]
          i -> [w288]
          n119 = Index Array(array=w287, index=w288) -> (element=w286:cluster{"Card Handle":u64, "Error Code":u32})
          n120 = call "spcm_vClose.vi"("Card Info In"=w286) -> ()  [unwired: 7 in]
        }
        n121 = Enqueue Element(queue=w285, element=element_states_io_sync."Quit", error in (no error)=w284) -> (error out=w283:errorcluster)  [unwired: 1 in, 2 out]
      }
      frame "Quit" {
      }
    }
  }
  n122 = while {
    tunnel: w5 -> [w302]
    tunnel: [w301] -> w4
    tunnel: w3 -> [w300]
    tunnel: [w299] -> w2
    stop <- w298 stop-if-true
    n123 = event shown="[1] \"Stop Button\": Value Change" {
      selector: _ -> [_ _ _]
      dyn-events: _ -> [_ _ _]
      timeout: _ -> [_ _ _]
      tunnel: w302 -> [w308 w313 w319]
      tunnel: [w307 w312 w318] -> w301
      tunnel: w300 -> [w306 w311 w317]
      tunnel: [w305 w310 w316] -> w299
      tunnel: [_ _ TRUE] -> w298
      event "Singleshot Button": Value Change {
        n124 = event-data() -> ()  [unwired: 1 in, 1 out]
        n125 = Enqueue Element(queue=w308, element=element_states_io_sync."Write Setup", error in (no error)=w306) -> (queue out=w307:refnum<queue>, error out=w305:errorcluster)  [unwired: 1 in, 1 out]
      }
      event "Stop Button": Value Change {
        n126 = event-data() -> ()  [unwired: 1 in, 1 out]
        n127 = Enqueue Element(queue=w313, element=element_states_io_sync."Stop", error in (no error)=w311) -> (queue out=w312:refnum<queue>, error out=w310:errorcluster)  [unwired: 1 in, 1 out]
      }
      event "Quit Button": Value Change {
        n128 = event-data() -> ()  [unwired: 1 in, 1 out]
        n129 = Enqueue Element(queue=w319, element=element_states_io_sync."Close Cards", error in (no error)=w317) -> (queue out=w318:refnum<queue>, error out=w316:errorcluster)  [unwired: 1 in, 1 out]
      }
    }
    n130 = Wait (ms)(milliseconds to wait=50) -> ()  [unwired: 1 out]
  }
  n131 = Merge Errors(w2, w1) -> (w6:errorcluster)
  n132 = Release Queue(queue=w4, error in (no error)=w6) -> ()  [unwired: 1 in, 3 out]
